vi "graphcleat.vi"() -> ()   [LabVIEW 2021]
panel:
  in  "stop":bool
  out "Waveform Graph":dynamicdata(graph)
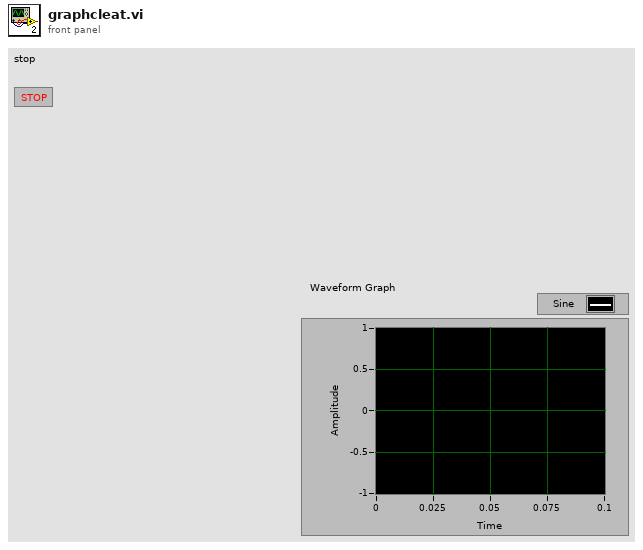
[diagram p1: front panel]
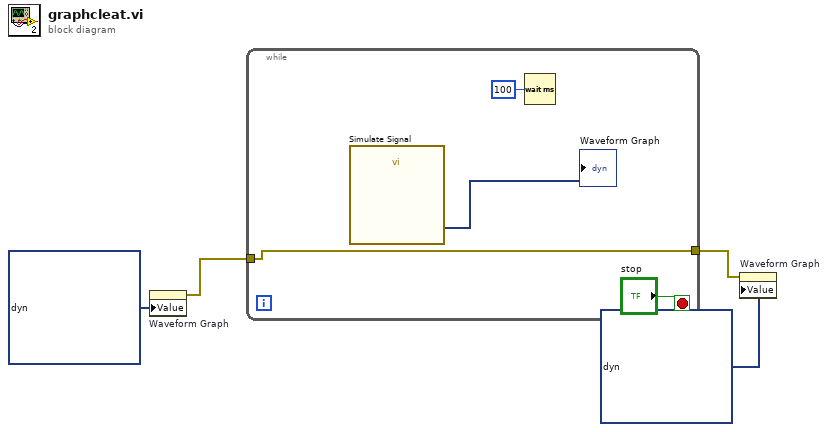
[diagram p0: block diagram]
diagram:
  n1 = property on="Waveform Graph" class="WFGraph (strict)"("Value"=dynamicdata [] ("Waveform Graph")) -> (error out=w3:errorcluster)  [unwired: 2 in, 1 out]
  n2 = while {
    tunnel: w3 -> [w5]
    tunnel: [w5] -> w2
    stop <- "stop" stop-if-true
    n3 = call "Simulate Signal"() -> ("Sine"=→"Waveform Graph":dynamicdata)  [unwired: 14 in, 1 out]
    n4 = Wait (ms)(milliseconds to wait=u32 100) -> ()  [unwired: 1 out]
  }
  n5 = property on="Waveform Graph" class="WFGraph (strict)"(error in=w2, "Value"=dynamicdata [] ("Waveform Graph")) -> ()  [unwired: 1 in, 2 out]
